vi "Picture Prompt.vi"(8 "error in (no error)":errorcluster, 10 "2D Picture 2":picture) -> (0 "error out":errorcluster)   [LabVIEW 2025]
panel:
  out "2D Picture":picture
  in  "OK Button":bool
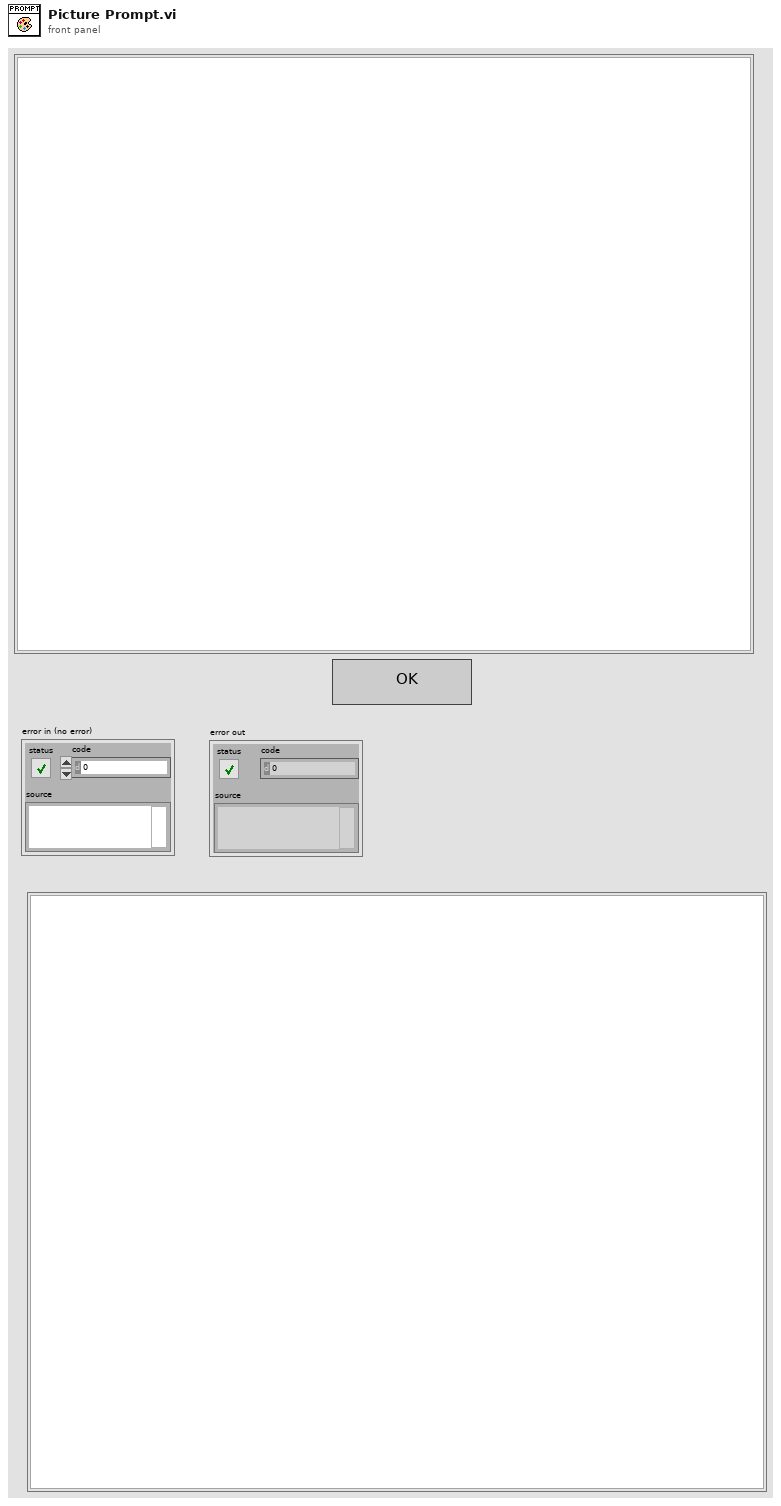
[diagram p1: front panel]
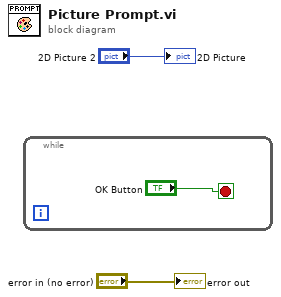
[diagram p0: block diagram]
diagram:
  n1 = while {
    stop <- "OK Button" stop-if-true
  }
  "error out" <- "error in (no error)"
  "2D Picture" <- "2D Picture 2"
